vi "Grow If Necessary.vi"(2 "number of additional datums (1)":i32=1, 3 "bytestream in":refnum<class "Bytestream.lvclass">) -> (1 "bytestream out":refnum<class "Bytestream.lvclass">)   [LabVIEW 2020, in "NI_Bytestream.lvlib" / "Bytestream.lvclass"]
uses:
  <vilib>/Array/Bytestream/Bytestream.lvclass
  <vilib>/Array/Bytestream/Bytestream.lvclass/Bytestream.ctl
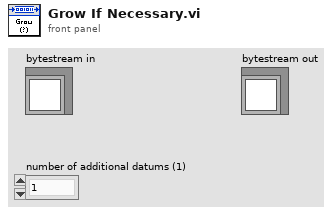
[diagram p1: front panel]
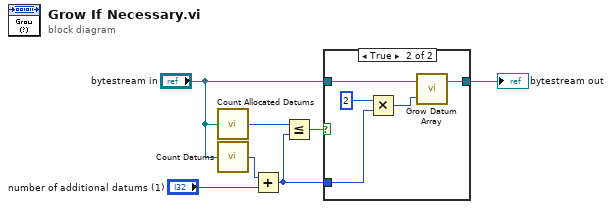
[diagram p0: block diagram]
diagram:
  n1 = call <vilib>:"Count Allocated Datums.vi"("bytestream"="bytestream in") -> ("datums"=w4:i32)
  n2 = call <vilib>:"Count Datums.vi"("bytestream"="bytestream in") -> ("datums"=w3:i32)
  n3 = Add(x=w3, y="number of additional datums (1)") -> (x+y=w1:i32)
  n4 = Less Or Equal?(x=w4, y=w1) -> (x <= y?=w5:bool)
  n5 = case shown="True" w5 {
    tunnel: "bytestream in" -> [w8 w13]
    tunnel: [w8 w12] -> w7
    tunnel: w1 -> [_ w9]
    frame False {
    }
    frame True {
      n6 = Multiply(x=2 ("y"), y=w9) -> (x*y=w10:i32)
      n7 = call <vilib>:"Grow Datum Array.vi"("size"=w10, "bytestream"=w13) -> ("bytestream out"=w12:refnum<class "Bytestream.lvclass">)  [unwired: 1 in]
    }
  }
  "bytestream out" <- w7
